vi "open.vi"(8 "error in (no error)":errorcluster caption="错误输入（无错误）", 11 "serial 输入":refnum<class "serial.lvclass">) -> (0 "error out":errorcluster caption="错误输出", 3 "serial 输出":refnum<class "serial.lvclass">)   [LabVIEW 2016, in "中水三立SQL数据传输.lvlib" / "serial.lvclass"]
uses:
  serial.lvclass
  <vilib>/Instr/_visa.llb/VISA Flush IO Buffer Mask.ctl
  data_inter/data_inter.lvclass/data_inter.ctl
  <vilib>/Instr/_visa.llb/VISA Configure Serial Port (Instr).vi
  data_inter/data_inter.lvclass
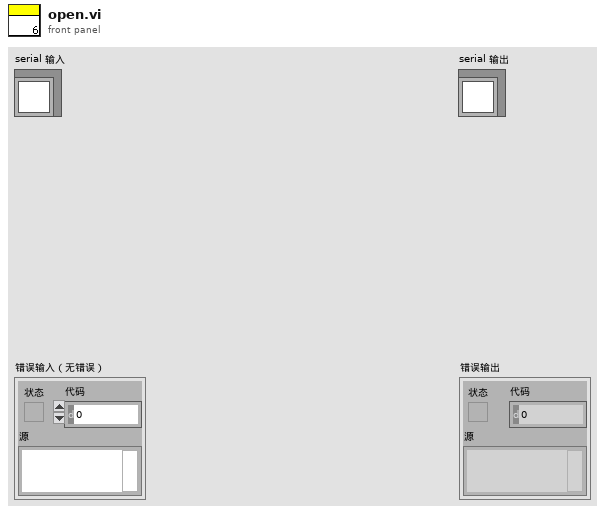
[diagram p1: front panel]
types:
  T1 = typedef "VISA Flush IO Buffer Mask.ctl" = u16
  T2 = cluster{"IP":string, "PORT":string, "VISA resource name":refnum<visa-resource-name>, "baud rate":u32}
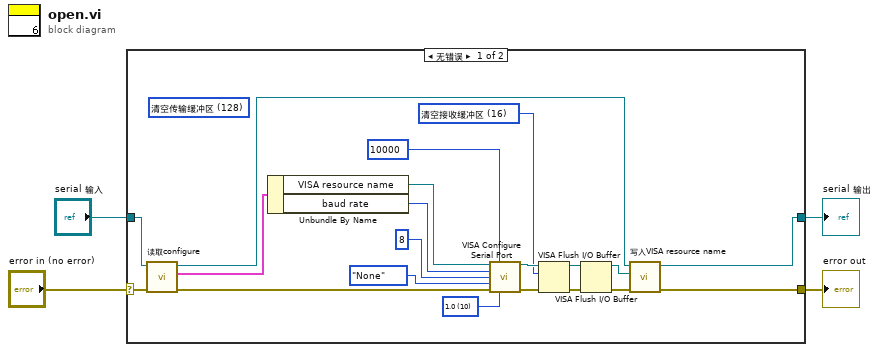
[diagram p0: block diagram]
diagram:
  n1 = case shown="无错误" "error in (no error)" {
    selector: "error in (no error)" -> [w22 w26]
    tunnel: [w5 w26] -> w3
    tunnel: "serial 输入" -> [w24 w25]
    tunnel: [w8 w25] -> w1
    frame No Error {
      w11 = u16 10 items=["1.0"=10, "1.5"=15, "2.0"=20] ("stop bits (10: 1 bit)")
      (unwired) T1 128 items=["清空接收缓冲区"=16, "向设备写入传输缓冲区"=32, "清空接收缓冲区（无I/O）"=64, "清空传输缓冲区"=128] ("Mask")
      w19 = T1 16 items=["清空接收缓冲区"=16, "向设备写入传输缓冲区"=32, "清空接收缓冲区（无I/O）"=64, "清空传输缓冲区"=128] ("Mask")
      n2 = call "读取configure.vi"("error in (no error)"=w22, "data_inter输入"=w24) -> ("error out"=w10:errorcluster, "configure"=w23:T2, "data_inter输出"=w9:refnum<class "serial.lvclass">)  [unwired: 7 in]
      n3 = Unbundle By Name(w23) -> ("VISA resource name"=w16:refnum<visa-resource-name>, "baud rate"=w15:u32)
      n4 = call-poly "VISA Configure Serial Port"("VISA resource name"=w16, "timeout (10sec)"=u32 10000, "baud rate (9600)"=w15, "data bits (8)"=u16 8, "parity (0:none)"=enum16{"None", "Odd", "Even", "Mark", "Space"}."None", "error in (no error)"=w10, "stop bits (10: 1 bit)"=w11) -> ("VISA resource name out"=w20:refnum<visa-resource-name>, "error out"=w21:errorcluster)  [unwired: 7 in]
      n5 = VISA Flush I/O Buffer(VISA resource name=w20, mask (16)=w19, error in (no error)=w21) -> (VISA resource name out=w17:refnum<visa-resource-name>, error out=w18:errorcluster)
      n6 = VISA Flush I/O Buffer(VISA resource name=w17, error in (no error)=w18) -> (VISA resource name out=w7:refnum<visa-resource-name>, error out=w6:errorcluster)  [unwired: 1 in]
      n7 = call-dynamic "写入VISA resource name.vi"("error in (no error)"=w6, "VISA resource name"=w7, "data_inter输入"=w9) -> ("error out"=w5:errorcluster, "data_inter输出"=w8:refnum<class "serial.lvclass">)  [unwired: 7 in]
    }
    frame Error {
    }
  }
  "error out" <- w3
  "serial 输出" <- w1
